vi "Séquencement.vi"() -> ()   [LabVIEW 2014]
panel:
  out "Horloge en 1/10 eme s":i32
  in  "Fin de  2eme etape":bool
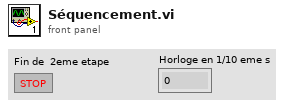
[diagram p1: front panel]
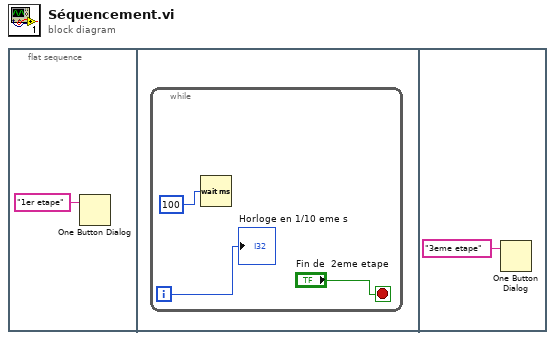
[diagram p0: block diagram]
diagram:
  n1 = flat-sequence {
    frame #0 {
      n2 = One Button Dialog(message="1er etape") -> ()  [unwired: 1 in, 1 out]
    }
    frame #1 {
      n3 = while {
        i -> [w2]
        stop <- "Fin de  2eme etape" stop-if-true
        n4 = Wait (ms)(milliseconds to wait=100) -> ()  [unwired: 1 out]
        "Horloge en 1/10 eme s" <- w2
      }
    }
    frame #2 {
      n5 = One Button Dialog(message="3eme etape") -> ()  [unwired: 1 in, 1 out]
    }
  }
